vi "Get System Channels refs.vi"(8 "error in (no error)":errorcluster, 11 "Item Ref in":T1 format="%.0x") -> (0 "error out":errorcluster, 2 "System Channel Refs":T1[](array[typedef]) format="%.0x", 3 "Item Ref out":T1 format="%.0x")   [LabVIEW 2019, in "Telemetry Engine.lvlib"]
uses:
  Telemetry Engine.lvlib
  <vilib>/NI VeriStand/Custom Device API/Custom Device Item Ref.ctl
  <vilib>/NI VeriStand/Custom Device Tools/Custom Device Utility Library/Custom Device Utility Library.lvlib
  <vilib>/NI VeriStand/Custom Device API/Custom Device API.lvlib
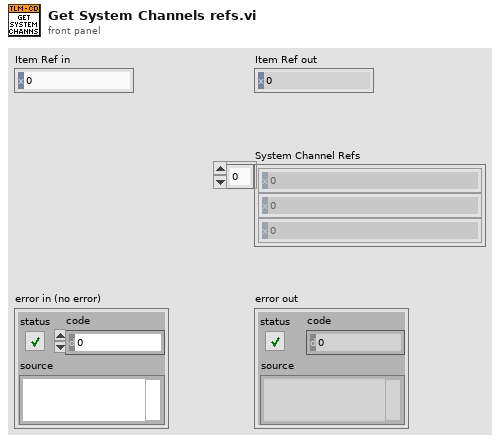
[diagram p1: front panel]
types:
  T1 = typedef "Custom Device API.lvlib/Custom Device Item Ref.ctl" = u64
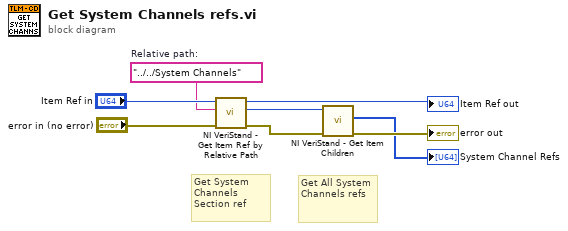
[diagram p0: block diagram]
diagram:
  w4 = "../../System Channels"  # Relative path:
  # "Get All System Channels refs"
  # "Get System Channels Section ref"
  n1 = call <vilib>:"NI VeriStand - Get Item Ref by Relative Path.vi"("error in"="error in (no error)", "Relative Item Path"=w4, "Section Ref in"="Item Ref in") -> ("error out"=w5:errorcluster, "Item Ref"=w3:T1, "Section Ref out"=→"Item Ref out":T1)  [unwired: 5 in, 1 out]
  n2 = call <vilib>:"NI VeriStand - Get Item Children.vi"("error in (no error)"=w5, "Item Ref in"=w3) -> ("error out"=→"error out":errorcluster, "Child Refs"=→"System Channel Refs":T1[])  [unwired: 6 in, 2 out]
